vi "ZCAN_Start_CAN.vi"(6 "abitbaud":u32, 7 "dbitbaud":u32, 8 "error in (no error)":errorcluster, 9 "ResistanceEnable":u32=1, 10 "device_hande":u32, 11 "can_index":u32) -> (0 "error out":errorcluster, 2 "startcan_success?":bool, 3 "can_index_handle(out)":u32)   [LabVIEW 2020, in "zlgcan.lvlib"]
uses:
  zlgcan.lvlib
  data_type/ZCAN_InitCAN_setting_USBCANFD.ctl
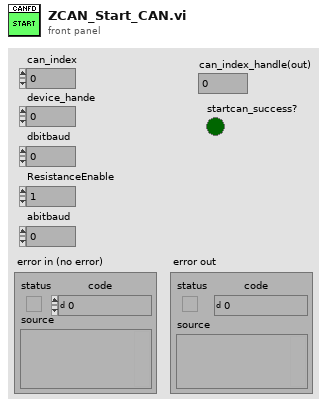
[diagram p1: front panel]
types:
  T1 = typedef "zlgcan.lvlib/ZCAN_InitCAN_setting_USBCANFD.ctl" = cluster{"abitbaud":u32, "dbitbaud":u32, "baud_rate_custom？":bool, "RateCustom":string, "mode":u8}
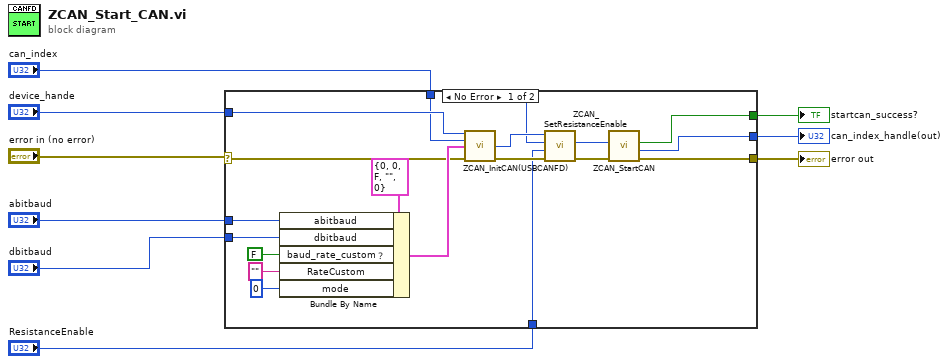
[diagram p0: block diagram]
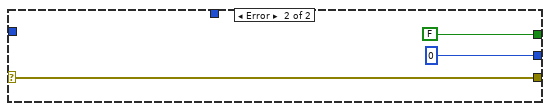
[diagram p2: hidden frame]
diagram:
  n1 = case shown="No Error" "error in (no error)" {
    selector: "error in (no error)" -> [w11 w30]
    tunnel: [w23 FALSE ("startcan_success?")] -> w9
    tunnel: "abitbaud" -> [w22 _]
    tunnel: "dbitbaud" -> [w21 _]
    tunnel: [w17 u32 0 ("can_index_handle(out)")] -> w6
    tunnel: "ResistanceEnable" -> [w16 _]
    tunnel: "device_hande" -> [w15 _]
    tunnel: "can_index" -> [w13 _]
    tunnel: [w10 w30] -> w1
    frame No Error {
      n2 = Bundle By Name(cluster=T1 {"abitbaud"=0, "dbitbaud"=0, "baud_rate_custom？"=FALSE, "RateCustom"="", "mode"=0} ("ZCAN_InitCAN_Setting_USBCANFD"), "abitbaud"=w22, "dbitbaud"=w21, "baud_rate_custom？"=FALSE, "RateCustom"="", "mode"=u8 0) -> (w24:T1)
      n3 = call "ZCAN_InitCAN(USBCANFD).vi"("device_hande"=w15, "can_index"=w13, "ZCAN_InitCAN_Setting_USBCANFD"=w24, "error in (no error)"=w11) -> ("can_index_handle"=w14:u32, "error out"=w27:errorcluster)  [unwired: 10 in]
      n4 = call "ZCAN_SetResistanceEnable.vi"("error in (no error)"=w27, "enable"=w16, "can_index"=w13, "can_index_handle"=w14) -> ("error out"=w26:errorcluster, "can_index_handle(out)"=w12:u32)  [unwired: 6 in]
      n5 = call "ZCAN_StartCAN.vi"("error in (no error)"=w26, "can_index_handle"=w12) -> ("error out"=w10:errorcluster, "can_index_handle(out)"=w17:u32, "startcan_success?"=w23:bool)  [unwired: 7 in]
    }
    frame Error {
    }
  }
  "startcan_success?" <- w9
  "can_index_handle(out)" <- w6
  "error out" <- w1
